vi "GetLifetimeOfDecay.vi"(0 "F2-channel":u8=1, 2 "decay":u32[][](array[numeric]), 5 "tauimage":bool) -> (8 "SpotProperties":T1 {"F2-Value overall" format="%.2f"; "tauerror" format="%.2f"; "Lifetime[ns]" format="%.2f"; "F2-Value TAC" format="%.2f"})   [LabVIEW 2009]
uses:
  spotproperties.ctl
panel:
  out "subarray":u32[](array[numeric])
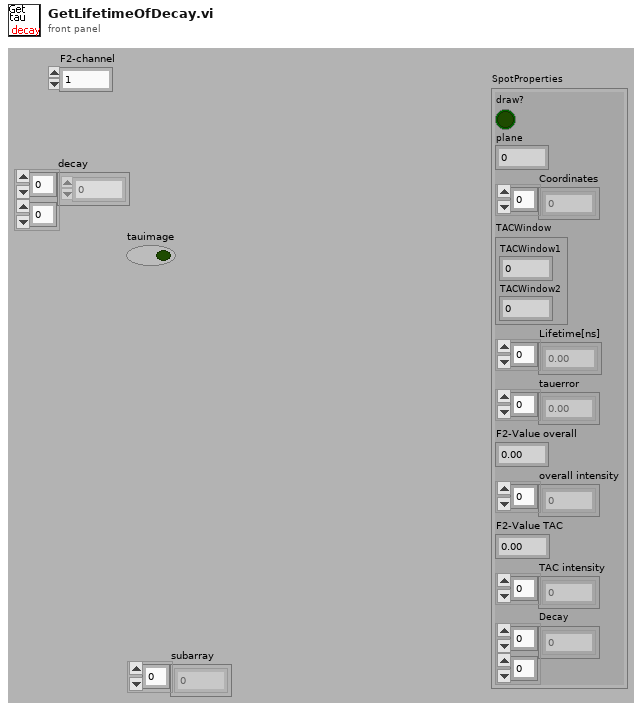
[diagram p1: front panel]
types:
  T1 = typedef "spotproperties.ctl" = cluster{"draw?":bool, "plane":u32, "Coordinates":i32[], "TACWindow":cluster{"TACWindow1":i32, "TACWindow2":i32}, "Lifetime[ns]":ext[], "tauerror":dbl[], "F2-Value overall":dbl, "overall intensity":u32[], "F2-Value TAC":dbl, "TAC intensity":u32[], "Decay":u32[][]}
  T2 = cluster{"CursorPos x1 out":i32, "CursorPos x0 out":i32}
  T3 = cluster{"CursorPos x1 out":dbl, "CursorPos x0 out":dbl}
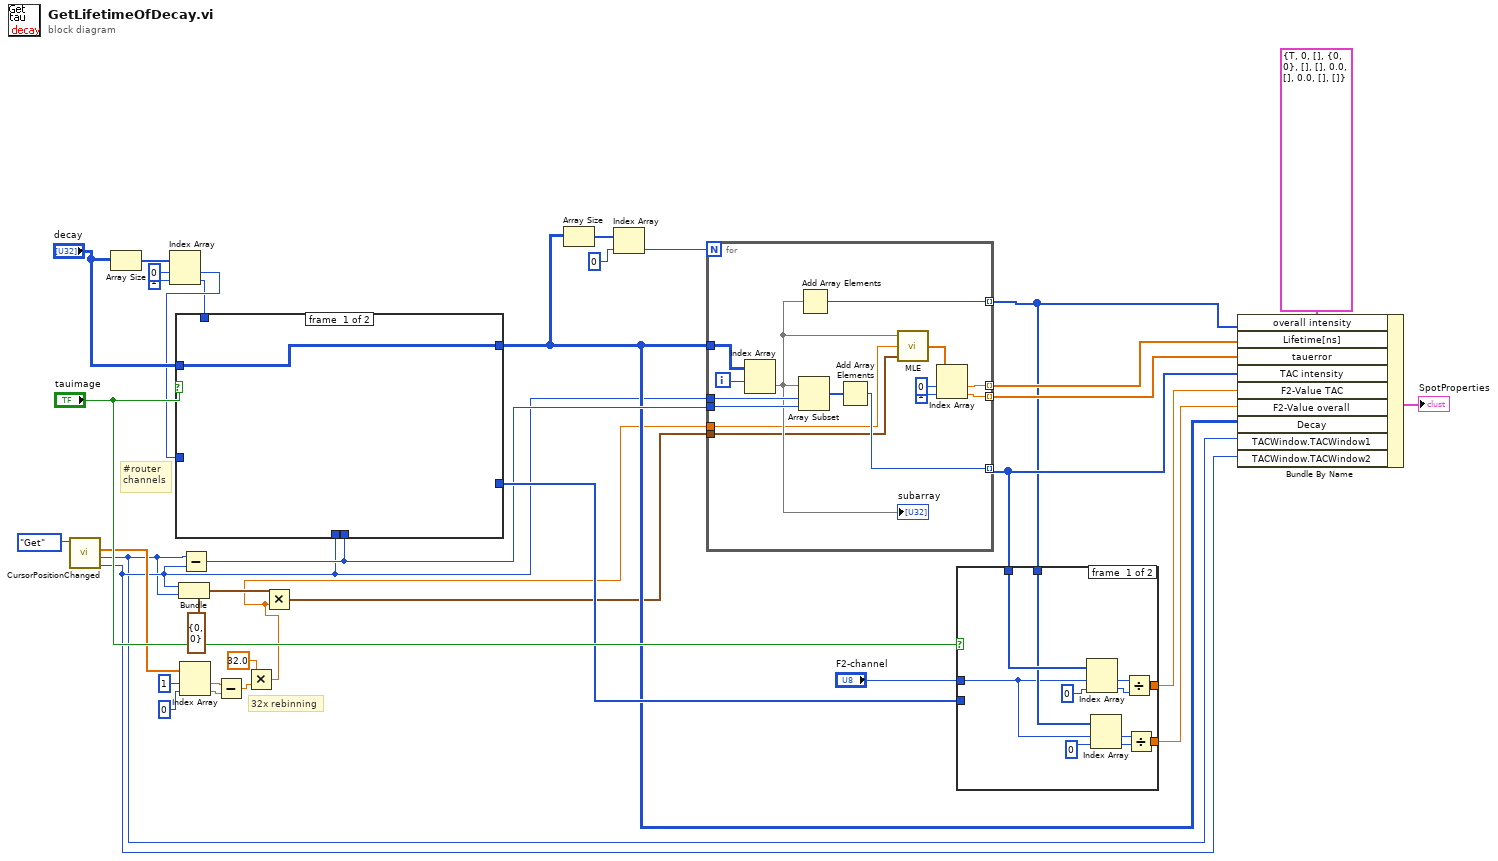
[diagram p0: block diagram]
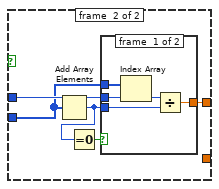
[diagram p2: hidden frame]
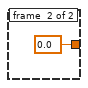
[diagram p3: hidden frame]
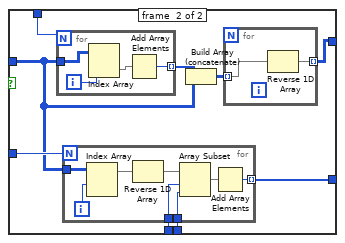
[diagram p4: hidden frame]
diagram:
  # "32x rebinning"
  # "#router \nchannels"
  n1 = call "CursorPositionChanged.vi"("action"=enum16{"Check", "Get"}."Get" ("Enum")) -> ("CursorPos min out"=w5:u16, "CursorPos max out"=w4:u16, "x-values out"=w12:dbl[])  [unwired: 3 in, 1 out]
  n2 = Array Size(array="decay") -> (size(s)=w34:i32[])
  n3 = Index Array(array=w34, index #1=0 ("index"), index #2=1 ("index")) -> (element #1=w29:i32, element #2=w19:i32)
  n4 = Bundle(cluster=T2 {"CursorPos x1 out"=0, "CursorPos x0 out"=0}, "CursorPos x1 out"=w5, "CursorPos x0 out"=w4) -> (w7:T2)
  n5 = Index Array(array=w12, index #1=1 ("index"), index #2=0 ("index")) -> (element #1=w8:dbl, element #2=w9:dbl)
  n6 = Subtract(x=w4, y=w5) -> (x-y=w18:u16)
  n7 = case shown="False" "tauimage" {
    tunnel: "decay" -> [w37 w40]
    tunnel: [w37 w39] -> w17
    tunnel: w5 -> [_ w46]
    tunnel: w18 -> [_ w45]
    tunnel: [_ w44] -> w31
    tunnel: w29 -> [_ w43]
    tunnel: w19 -> [_ w42]
    frame #0 {
    }
    frame #1 {
      n8 = for {
        N: w42 -> [_]
        tunnel: w40 -> [w60]
        tunnel: [w57] -> w41 mode=indexing
        i -> [w59]
        n9 = Index Array(array=w60, index (col)=w59) -> (element=w58:u32[])  [unwired: 1 in]
        n10 = Add Array Elements(numeric array=w58) -> (sum=w57:u32)
      }
      n11 = for {
        N: w43 -> [_]
        tunnel: w40 -> [w56]
        tunnel: w46 -> [w53]
        tunnel: w45 -> [w52]
        tunnel: [w50] -> w44 mode=indexing
        i -> [w55]
        n12 = Index Array(array=w56, index (row)=w55) -> (element=w54:u32[])  [unwired: 1 in]
        n13 = Reverse 1D Array(array=w54) -> (reversed array=w49:u32[])
        n14 = Array Subset(array=w49, index=w53, length=w52) -> (w51:u32[])
        n15 = Add Array Elements(numeric array=w51) -> (sum=w50:u32)
      }
      n16 = Build Array (concatenate)(w41, w40) -> (w38:u32[][])
      n17 = for {
        tunnel: [w48] -> w39 mode=indexing
        tunnel: w38 -> [w47] mode=indexing
        n18 = Reverse 1D Array(array=w47) -> (reversed array=w48:u32[])
      }
    }
  }
  n19 = Subtract(x=w8, y=w9) -> (x-y=w3:dbl)
  n20 = Multiply(x=32.0, y=w3) -> (x*y=w1:dbl)
  n21 = Multiply(x=w7, y=w1) -> (x*y=w6:T3)
  n22 = Array Size(array=w17) -> (size(s)=w16:i32[])
  n23 = Index Array(array=w16, index=0) -> (element=w14:i32)
  n24 = for {
    N: w14 -> [_]
    tunnel: [w66] -> w22 mode=indexing
    tunnel: [w75] -> w21 mode=indexing
    tunnel: w17 -> [w74]
    tunnel: [w65] -> w23 mode=indexing
    tunnel: w5 -> [w71]
    tunnel: w18 -> [w72]
    tunnel: [w70] -> w24 mode=indexing
    tunnel: w6 -> [w61]
    tunnel: w1 -> [w62]
    i -> [w73]
    n25 = Index Array(array=w74, index (row)=w73) -> (element=w63:u32[])  [unwired: 1 in]
    "subarray" <- w63
    n26 = Array Subset(array=w63, index=w71, length=w72) -> (w69:u32[])
    n27 = Add Array Elements(numeric array=w63) -> (sum=w75:u32)
    n28 = Add Array Elements(numeric array=w69) -> (sum=w70:u32)
    n29 = call "MLE.vi"("input range"=w61, "channel width (ns)"=w62, "lifetime histograms"=w63) -> ("lifetime (ns)"=w64:dbl[])
    n30 = Index Array(array=w64, index #1=0 ("index"), index #2=1 ("index")) -> (element #1=w66:dbl, element #2=w65:dbl)
  }
  n31 = case shown="True" "tauimage" {
    tunnel: [w86 w91] -> w25
    tunnel: "F2-channel" -> [w79 w90]
    tunnel: w24 -> [w84 _]
    tunnel: w31 -> [_ w89]
    tunnel: w21 -> [w80 _]
    tunnel: [w76 _] -> w26
    frame #0 {
      n32 = Index Array(array=w84, index #1=w79, index #2=0 ("index")) -> (element #1=w85:u32, element #2=w82:u32)
      n33 = Index Array(array=w80, index #1=w79, index #2=0 ("index")) -> (element #1=w78:u32, element #2=w77:u32)
      n34 = Divide(x=w85, y=w82) -> (x/y=w86:dbl)
      n35 = Divide(x=w78, y=w77) -> (x/y=w76:dbl)
    }
    frame #1 {
      n36 = Add Array Elements(numeric array=w89) -> (sum=w87:u32)
      n37 = Equal To 0?(x=w87) -> (x = 0?=w88:bool)
      n38 = case shown="True" w88 {
        tunnel: [w96 0.0] -> w91
        tunnel: w90 -> [w94 _]
        tunnel: w87 -> [w93 _]
        tunnel: w89 -> [w92 _]
        frame #0 {
          n39 = Index Array(array=w92, index=w94) -> (element=w95:u32)
          n40 = Divide(x=w95, y=w93) -> (x/y=w96:dbl)
        }
        frame #1 {
        }
      }
    }
  }
  n41 = Bundle By Name(cluster=T1 {"draw?"=TRUE, "plane"=0, "Coordinates"=[], "TACWindow"={"TACWindow1"=0, "TACWindow2"=0}, "Lifetime[ns]"=[], "tauerror"=[], "F2-Value overall"=0.0, "overall intensity"=[], "F2-Value TAC"=0.0, "TAC intensity"=[], "Decay"=[]} ("SpotProperties"), "overall intensity"=w21, "Lifetime[ns]"=w22, "tauerror"=w23, "TAC intensity"=w24, "F2-Value TAC"=w25, "F2-Value overall"=w26, "Decay"=w17, "TACWindow.TACWindow1"=w4, "TACWindow.TACWindow2"=w5) -> (→"SpotProperties":T1)
